vi "digWaveFromPlatData_Manual.vi"() -> ()   [LabVIEW 2017]
uses:
  <vilib>/imath/engines/lvmath2/RunTimeEngine/BuiltInFunctions/length/NIMS_length(GV).vi
  <instcachedir>/0/NIMS_length(GV)_08A3D13377FD4E4B96F5795FBF3698FA.lvgen/NIMS_length(GV)_08A3D13377FD4E4B96F5795FBF3698FA_003.vi
  <vilib>/imath/engines/lvmath2/RunTimeEngine/BuiltInFunctions/repeatmx/NIMS_repeatmx(GM, I32, I32).vi
  <instcachedir>/0/NIMS_repeatmx(GM, I32, I32)_8EDBB852F26742A48D04758F158AC943.lvgen/NIMS_repeatmx(GM, I32, I32)_8EDBB852F26742A48D04758F158AC943_004.vi
  <vilib>/imath/engines/lvmath2/RunTimeEngine/RowToken/NIMS_RowToken_SorRV_M.vi
  <instcachedir>/0/NIMS_RowToken_SorRV_M_997882E9B890466D9AE38E5C4E8B9D70.lvgen/NIMS_RowToken_SorRV_M_997882E9B890466D9AE38E5C4E8B9D70_000.vi
  <vilib>/imath/engines/lvmath2/RunTimeEngine/ErrorHandling/NIMS_Create Error From Enums.vi
  <vilib>/imath/engines/lvmath2/RunTimeEngine/BuiltInFunctions/mirrorh/NIMS_mirrorh(GRowV).vi
  <instcachedir>/0/NIMS_mirrorh(GRowV)_B6A8CC4EAFBA4F9A82A59460D67BDFF0.lvgen/NIMS_mirrorh(GRowV)_B6A8CC4EAFBA4F9A82A59460D67BDFF0_000.vi
  <vilib>/imath/engines/lvmath2/RunTimeEngine/MatrixToken/NIMS_MatrixToken_RV_RV.vi
  <instcachedir>/0/NIMS_MatrixToken_RV_RV_8B087EE0EE16477EBE1C341EABB504F3.lvgen/NIMS_MatrixToken_RV_RV_8B087EE0EE16477EBE1C341EABB504F3_002.vi
  <vilib>/imathl/engines/lvmath/Functions/Error Handling/Create Error.vi
  <vilib>/imath/engines/lvmath2/RunTimeEngine/IndexRead/NIMS M($).vi
  <instcachedir>/0/NIMS M($)_82D1177398184AFB96A6AFB63C3C3F57.lvgen/NIMS M($)_82D1177398184AFB96A6AFB63C3C3F57_005.vi
  <vilib>/imath/engines/lvmath2/RunTimeEngine/MatrixToken/NIMS_MatrixToken_M_RV.vi
  <instcachedir>/0/NIMS_MatrixToken_M_RV_EE6E048DE0454E429C3E3ED099F2A9DF.lvgen/NIMS_MatrixToken_M_RV_EE6E048DE0454E429C3E3ED099F2A9DF_002.vi
  <vilib>/imath/engines/lvmath2/RunTimeEngine/NodeEndStatement/NIMS_NodeEndStatement_Output.vi
  <instcachedir>/0/NIMS_NodeEndStatement_Output_53EC0D466D134D7ABD903AC30B43404B.lvgen/NIMS_NodeEndStatement_Output_53EC0D466D134D7ABD903AC30B43404B_012.vi
  <vilib>/imath/engines/lvmath2/RunTimeEngine/ErrorHandling/NIMS_Finalize Error.vi
panel:
  in  "mazeDirection":string(combo)="clockwise"
  out "Digital Waveform Graph 3":digitalwaveform(graph)
  out "Digital Waveform Graph":digitalwaveform(graph)
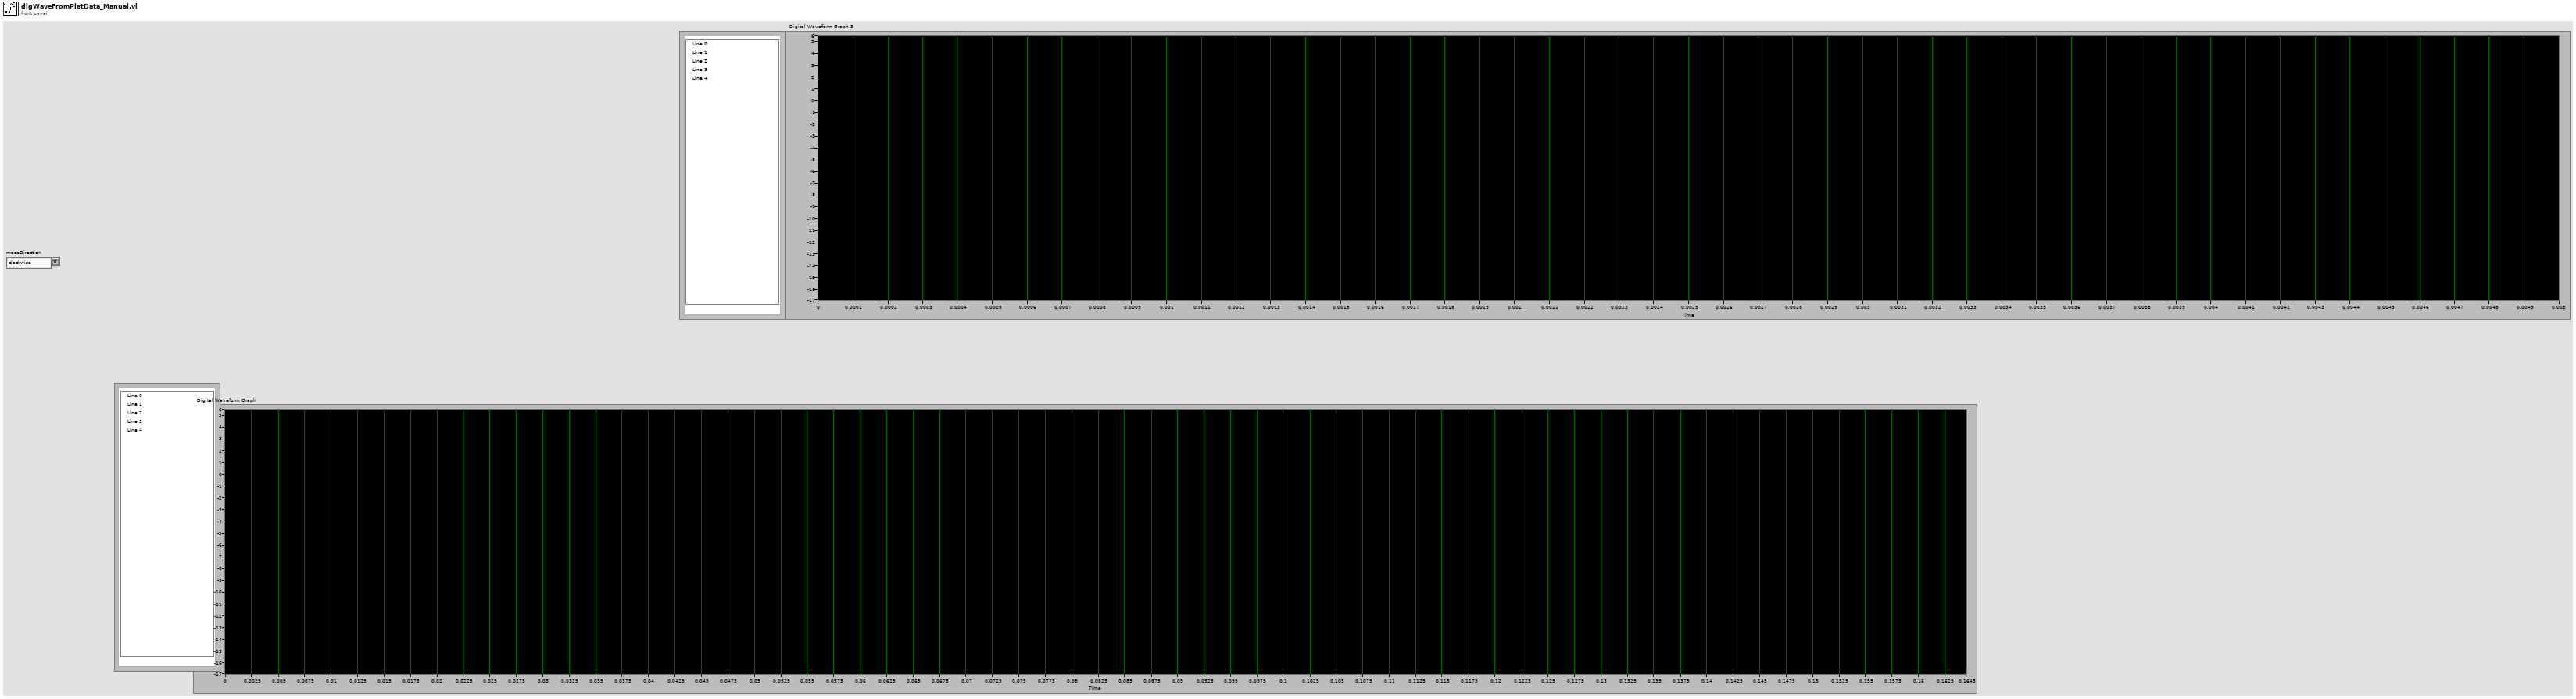
[diagram p1: front panel]
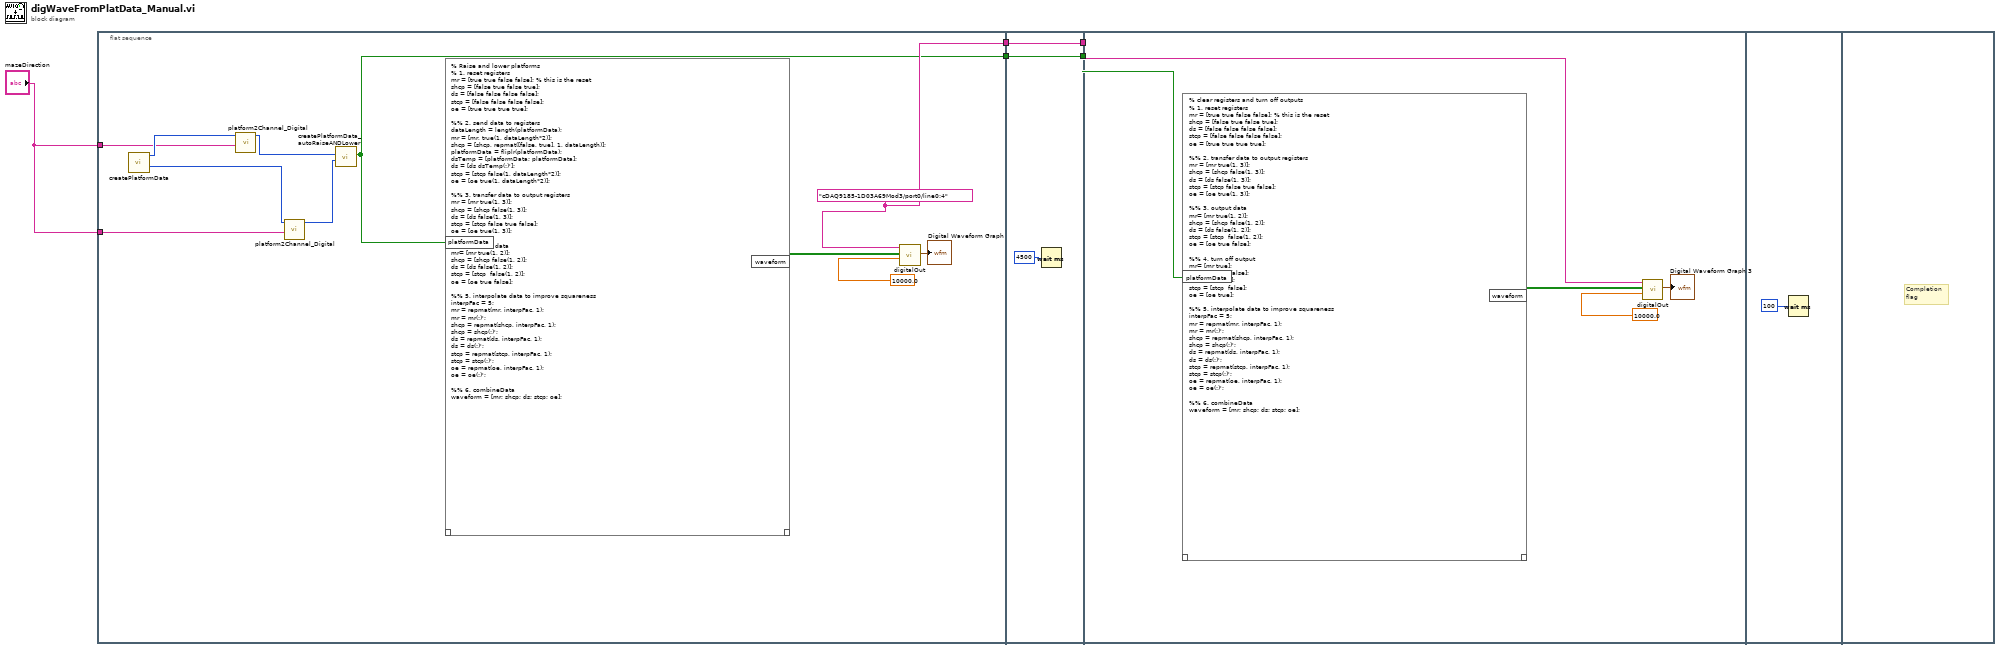
[diagram p0: block diagram]
diagram:
  n1 = flat-sequence {
    tunnel: [w12] -> w5
    tunnel: [w13] -> w4
    tunnel: "mazeDirection" -> [w7]
    tunnel: "mazeDirection" -> [w6]
    tunnel: w5 -> [w490]
    tunnel: [w490] -> w3
    tunnel: w4 -> [w489]
    tunnel: [w489] -> w2
    tunnel: w3 -> [w496]
    tunnel: w2 -> [w492]
    frame #0 {
      w13 = tag "cDAQ9185-1D03A69Mod3/port0/line0:4" ("lines")
      n2 = call "createPlatformData.vi"() -> ("platforms to \nlower"=w8:i32[], "platforms to \nraise"=w9:i32[])  [unwired: 10 in]
      n3 = call "platform2Channel_Digital.vi"("mazeDirection"=w7, "Platforms"=w9) -> ("channels"=w11:i32[])  [unwired: 9 in]
      n4 = call "platform2Channel_Digital.vi"("mazeDirection"=w6, "Platforms"=w8) -> ("channels"=w10:i32[])  [unwired: 9 in]
      n5 = call "createPlatformData_autoRaiseANDLower.vi"("Plaforms to raise"=w11, "Plaforms to lower"=w10) -> ("platformData"=w12:bool[])  [unwired: 8 in]
      n6 = mathscript code="% Raise and lower platforms\n% 1. reset registers\nmr = [true true false false]; % this is the reset\nshcp = [false true false true];\nds = [false false false false];\nstcp = [false false false false];\noe = [true true true true];\n\n%% 2. send data to registers\ndataLength = length(platformData); \nmr = [mr, true(1, dataLength*2)];\nshcp = [shcp, repmat([false, true], 1, dataLength)];\nplatformData = fliplr(platformData);\ndsTemp = [platformData; platformData];\nds = [ds dsTemp(:)'];\nstcp = [stcp false(1, dataLength*2)];\noe = [oe true(1, dataLength*2)];\n\n%% 3. transfer data to output registers\nmr = [mr true(1, 3)];\nshcp = [shcp false(1, 3)];\nds = [ds false(1, 3)];\nstcp = [stcp false true false];\noe = [oe true(1, 3)];\n\n%% 4. output data\nmr= [mr true(1, 2)];\nshcp = [shcp false(1, 2)];\nds = [ds false(1, 2)];\nstcp = [stcp  false(1, 2)];\noe = [oe true false];\n\n%% 5. interpolate data to improve squareness\ninterpFac = 5;\nmr = repmat(mr, interpFac, 1);\nmr = mr(:)';\nshcp = repmat(shcp, interpFac, 1);\nshcp = shcp(:)';\nds = repmat(ds, interpFac, 1);\nds = ds(:)';\nstcp = repmat(stcp, interpFac, 1);\nstcp = stcp(:)';\noe = repmat(oe, interpFac, 1);\noe = oe(:)';\n\n%% 6. combineData\nwaveform = [mr; shcp; ds; stcp; oe];"("platformData"=w12) -> ("waveform"=w15:bool[][])  [unwired: 1 in, 1 out]
      n7 = call "digitalOut.vi"("rate"=10000.0, "waveform"=w15, "lines"=w13) -> ("digital waveform"=→"Digital Waveform Graph":digitalwaveform)  [unwired: 8 in]
    }
    frame #1 {
      n8 = Wait (ms)(milliseconds to wait=4500) -> ()  [unwired: 1 out]
    }
    frame #2 {
      n9 = mathscript code="% clear registers and turn off outputs\n% 1. reset registers\nmr = [true true false false]; % this is the reset\nshcp = [false true false true];\nds = [false false false false];\nstcp = [false false false false];\noe = [true true true true];\n\n%% 2. transfer data to output registers\nmr = [mr true(1, 3)];\nshcp = [shcp false(1, 3)];\nds = [ds false(1, 3)];\nstcp = [stcp false true false];\noe = [oe true(1, 3)];\n\n%% 3. output data \nmr= [mr true(1, 2)];\nshcp = [shcp false(1, 2)];\nds = [ds false(1, 2)];\nstcp = [stcp  false(1, 2)];\noe = [oe true false];\n\n%% 4. turn off output\nmr= [mr true];\nshcp = [shcp false];\nds = [ds false];\nstcp = [stcp  false];\noe = [oe true];\n\n%% 5. interpolate data to improve squareness\ninterpFac = 5;\nmr = repmat(mr, interpFac, 1);\nmr = mr(:)';\nshcp = repmat(shcp, interpFac, 1);\nshcp = shcp(:)';\nds = repmat(ds, interpFac, 1);\nds = ds(:)';\nstcp = repmat(stcp, interpFac, 1);\nstcp = stcp(:)';\noe = repmat(oe, interpFac, 1);\noe = oe(:)';\n\n%% 6. combineData\nwaveform = [mr; shcp; ds; stcp; oe];"("platformData"=w496) -> ("waveform"=w494:bool[][])  [unwired: 1 in, 1 out]
      n10 = call "digitalOut.vi"("rate"=10000.0, "waveform"=w494, "lines"=w492) -> ("digital waveform"=→"Digital Waveform Graph 3":digitalwaveform)  [unwired: 8 in]
    }
    frame #3 {
      n11 = Wait (ms)(milliseconds to wait=100) -> ()  [unwired: 1 out]
    }
    frame #4 {
      # "Completion\nflag"
    }
  }
